vi "Z900_navX_Set_ZeroDisplacement.vi"(8 "error in (no error)":errorcluster, 10 "Zero Vector":T1={"X"=TRUE, "Y"=TRUE, "Z"=TRUE}, 11 "navX Device":T2={"Interface"={"Protocol"=enum."SERIAL", "Update Rate (4Hz-100Hz)"=4, "navX Open TypeDef"=variant}, "Notify Packet"=refnum, "Loop VI Refnum"=refnum, "Ready to Close Occurrence Refnum"=refnum} {"Interface"."Update Rate (4Hz-100Hz)" min=4 max=60 step=1}) -> (0 "error out":errorcluster, 3 "navX Device":T2={"Interface"={"Protocol"=enum."SERIAL", "Update Rate (4Hz-100Hz)"=4, "navX Open TypeDef"=variant}, "Notify Packet"=refnum, "Loop VI Refnum"=refnum, "Ready to Close Occurrence Refnum"=refnum} {"Interface"."Update Rate (4Hz-100Hz)" min=4 max=60 step=1})   [LabVIEW 2016, in "navX Library v2.lvlib"]
uses:
  navX Library v2.lvlib
  TypeDefs/Z900_navX_DeviceTypeDef.ctl
  TypeDefs/Z900_navX_ProtocolTypeDef.ctl
  TypeDefs/Z900_navX_NotifyPacketTypeDef.ctl
  TypeDefs/Z900_navX_ActionTypeDef.ctl
  TypeDefs/Z900_navX_ZeroVectorTypeDef.ctl
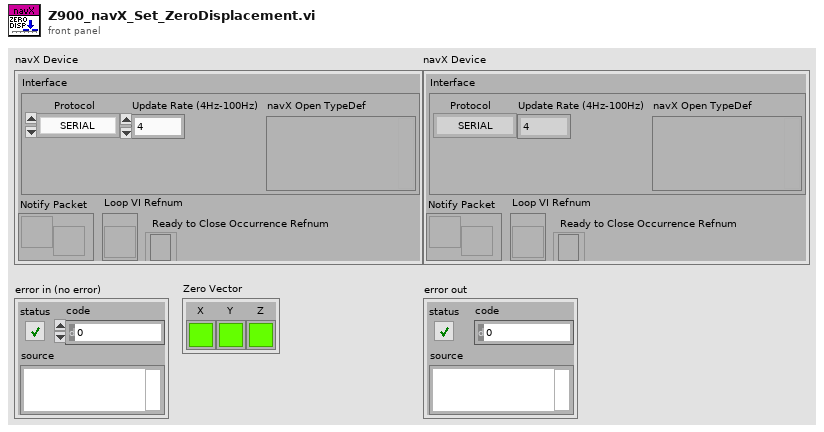
[diagram p1: front panel]
types:
  T1 = typedef "navX Library v2.lvlib/Z900_navX_ZeroVectorTypeDef.ctl" = cluster{"X":bool, "Y":bool, "Z":bool}
  T2 = typedef "navX Library v2.lvlib/Z900_navX_DeviceTypeDef.ctl" = cluster{"Interface":cluster{"Protocol":T3, "Update Rate (4Hz-100Hz)":u8, "navX Open TypeDef":variant}, "Notify Packet":refnum<notifier>, "Loop VI Refnum":refnum<vi>, "Ready to Close Occurrence Refnum":refnum<k4>}
  T3 = typedef "navX Library v2.lvlib/Z900_navX_ProtocolTypeDef.ctl" = enum16{"SERIAL", "I2C", "SPI"}
  T4 = typedef "navX Library v2.lvlib/Z900_navX_ActionTypeDef.ctl" = enum16{"None", "Halt", "Update Serial Protocol", "Zero-Yaw", "Zero-Displacement", "Zero-Velocity"}
  T5 = typedef "navX Library v2.lvlib/Z900_navX_NotifyPacketTypeDef.ctl" = cluster{"navX Action":T4, "Data":variant}
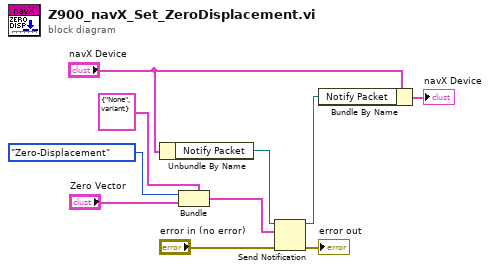
[diagram p0: block diagram]
diagram:
  n1 = Unbundle By Name("navX Device") -> ("Notify Packet"=w10:refnum<notifier>)
  n2 = Bundle(cluster=T5 {"navX Action"=enum."None", "Data"=variant} ("navX Notify Packet"), "navX Action"=Z900_navX_ActionTypeDef."Zero-Displacement", "Data"="Zero Vector") -> (w7:T5)
  n3 = Send Notification(notification=w7, notifier=w10, error in (no error)="error in (no error)") -> (notifier out=w9:refnum<notifier>, error out=→"error out":errorcluster)
  n4 = Bundle By Name(cluster="navX Device", "Notify Packet"=w9) -> (→"navX Device":T2)
